vi "Get Density v2 PN.vi"(2 "Timing SW trigger":tag="Dev1/port2/line7", 3 "Counter":tag="Dev1/ctr0", 4 "Device":tag="Dev1") -> (0 "Error":errorcluster, 1 "Density (kg/m^3)":dbl)   [LabVIEW 2011]
uses:
  <vilib>/DAQmx/read.llb/DAQmx Read (Digital Bool 1Line 1Point).vi
  <vilib>/DAQmx/create/channels.llb/DAQmx Create Channel (CI-Count Edges).vi
  <vilib>/DAQmx/create/channels.llb/DAQmx Create Channel (DI-Digital Input).vi
  <vilib>/DAQmx/read.llb/DAQmx Read (Counter U32 1Chan 1Samp).vi
panel:
  # "by Paul Nathan, 22/01/2012"
  # "Revisions:\nDate       Desc.      Auth.\nx               x               x"
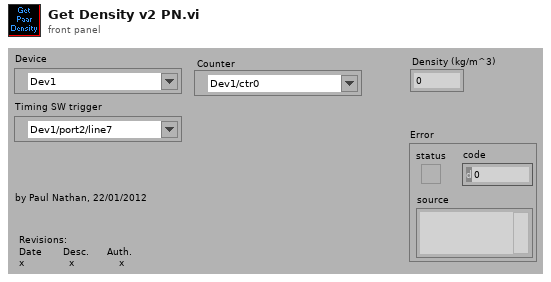
[diagram p1: front panel]
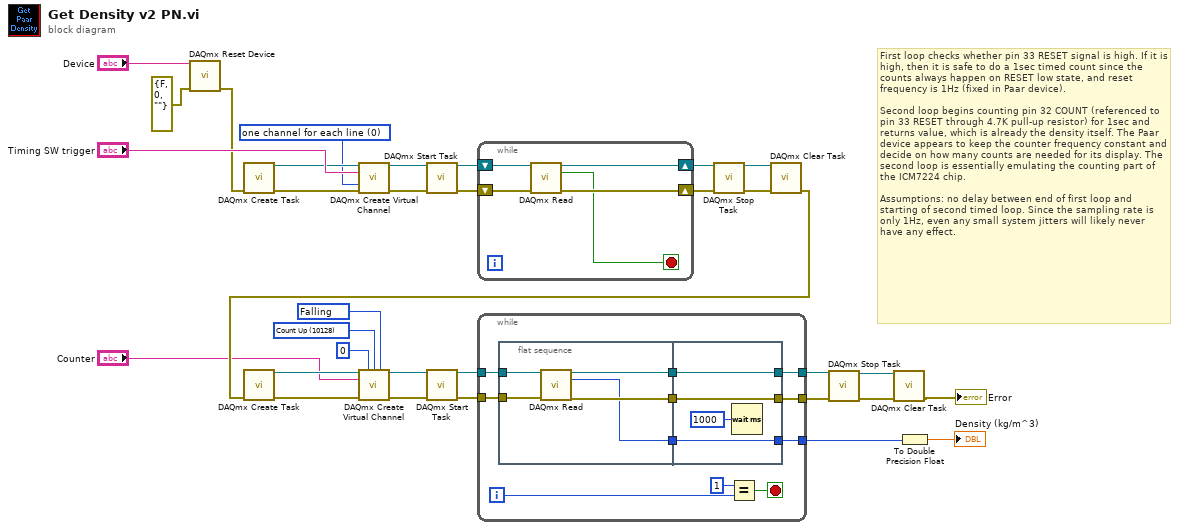
[diagram p0: block diagram]
diagram:
  w7 = 10171 items=["Rising"=10280, "Falling"=10171] ("edge")
  w6 = 10128 items=["Count Up"=10128, "Count Down"=10124, "Externally Controlled"=10326] ("count direction")
  w25 = 0 items=["one channel for each line", "one channel for all lines"] ("line grouping")
  # "First loop checks whether pin 33 RESET signal is high. If it is high, then it is safe to do a 1sec timed count since the counts always happen on RESET low state, and reset frequency is 1Hz (fixed in Paar device).\n\nSecond loop begins counting pin 32 COUNT (referenced to pin 33 RESET through 4.7K pull-up resistor) for 1sec and returns value, which is already the density itself. The Paar device appears to keep the counter frequency constant and decide on how many counts are needed for its display. The second loop is essentially emulating the counting part of the ICM7224 chip.\n\nAssumptions: no delay between end of first loop and starting of second timed loop. Since the sampling rate is only 1Hz, even any small system jitters will likely never have any effect."
  n1 = call <vilib>:"DAQmx Reset Device.vi"("device in"="Device", "error in"=errorcluster {"status"=FALSE, "code"=0, "source"=""}) -> ("error out"=w28:errorcluster)  [unwired: 13 in]
  n2 = call <vilib>:"DAQmx Create Task.vi"("error in"=w28) -> ("task out"=w26:refnum<k21>, "error out"=w23:errorcluster)  [unwired: 13 in]
  n3 = call-poly <vilib>:"DAQmx Create Virtual Channel.vi"("task in"=w26, "lines"="Timing SW trigger", "line grouping"=w25, "error in"=w23) -> ("task out"=w22:refnum<k21>, "error out"=w24:errorcluster)  [unwired: 10 in]
  n4 = call <vilib>:"DAQmx Start Task.vi"("task/channels in"=w22, "error in"=w24) -> ("task out"=w21:refnum<k21>, "error out"=w18:errorcluster)  [unwired: 12 in]
  n5 = while {
    shift-right: [w37] -> w16
    shift-left: w18 -> [w36]
    shift-right: [w35] -> w17
    shift-left: w21 -> [w38]
    stop <- w34 stop-if-true
    n6 = call-poly <vilib>:"DAQmx Read.vi"("task/channels in"=w38, "error in"=w36) -> ("task out"=w35:refnum<k21>, "data"=w34:bool, "error out"=w37:errorcluster)  [unwired: 11 in]
  }
  n7 = call <vilib>:"DAQmx Stop Task.vi"("task/channels in"=w17, "error in"=w16) -> ("task out"=w20:refnum<k21>, "error out"=w19:errorcluster)  [unwired: 12 in]
  n8 = call <vilib>:"DAQmx Clear Task.vi"("task in"=w20, "error in"=w19) -> ("error out"=w27:errorcluster)  [unwired: 13 in]
  n9 = call <vilib>:"DAQmx Create Task.vi"("error in"=w27) -> ("task out"=w3:refnum<k21>, "error out"=w1:errorcluster)  [unwired: 13 in]
  n10 = call-poly <vilib>:"DAQmx Create Virtual Channel.vi"("task in"=w3, "initial count"=u32 0, "count direction"=w6, "edge"=w7, "counter"="Counter", "error in"=w1) -> ("task out"=w8:refnum<k21>, "error out"=w9:errorcluster)  [unwired: 8 in]
  n11 = call <vilib>:"DAQmx Start Task.vi"("task/channels in"=w8, "error in"=w9) -> ("task out"=w14:refnum<k21>, "error out"=w15:errorcluster)  [unwired: 12 in]
  n12 = while {
    tunnel: w15 -> [w49]
    tunnel: w14 -> [w48]
    tunnel: [w47] -> w12
    tunnel: [w46] -> w13
    tunnel: [w42] -> w29
    i -> [w45]
    stop <- w43 stop-if-true
    n13 = flat-sequence {
      tunnel: w49 -> [w54]
      tunnel: w48 -> [w53]
      tunnel: [w52] -> w41
      tunnel: [w51] -> w40
      tunnel: [w50] -> w39
      tunnel: [w56] -> w42
      tunnel: [w57] -> w46
      tunnel: [w58] -> w47
      tunnel: w41 -> [w58]
      tunnel: w40 -> [w57]
      tunnel: w39 -> [w56]
      frame #0 {
        n14 = call-poly <vilib>:"DAQmx Read.vi"("task/channels in"=w53, "error in"=w54) -> ("task out"=w52:refnum<k21>, "data"=w50:u32, "error out"=w51:errorcluster)  [unwired: 11 in]
      }
      frame #1 {
        n15 = Wait (ms)(milliseconds to wait=u32 1000) -> ()  [unwired: 1 out]
      }
    }
    n16 = Equal?(x=1, y=w45) -> (x = y?=w43:bool)
  }
  n17 = call <vilib>:"DAQmx Stop Task.vi"("task/channels in"=w12, "error in"=w13) -> ("task out"=w11:refnum<k21>, "error out"=w10:errorcluster)  [unwired: 12 in]
  n18 = call <vilib>:"DAQmx Clear Task.vi"("task in"=w11, "error in"=w10) -> ("error out"=→"Error":errorcluster)  [unwired: 13 in]
  n19 = To Double Precision Float(number=w29) -> (double precision float=→"Density (kg/m^3)":dbl)
